vi "Local Tracking.vi"(4 "Offset Home 2 RCM":dbl[](array[numeric])=[0.0, 0.0, 0.0, 0.0], 5 "Trajectory Cluster":T1, 6 "PID Cluster":T4={"L1 to L4 PID Cluster"={"L1 PID Gains"={"Kp"=0.005, "Kd"=0.5, "Ki"=0.0005}, "L2 PID Gains"={"Kp"=0.01, "Kd"=1.0, "Ki"=0.005}, "L3 PID Gains"={"Kp"=0.05, "Kd"=1.0, "Ki"=0.0005}, "L4 PID Gains"={"Kp"=0.1, "Kd"=0.1, "Ki"=0.0005}}, "Stage PID Cluster"={"Stage Z PID"={"Kp"=0.0005, "Kd"=0.001, "Ki"=0.0}, "Stage Y PID"={"Kp"=0.0003, "Kd"=0.01, "Ki"=0.0}, "Stage X PID"={"Kp"=0.0003, "Kd"=0.01, "Ki"=0.0}}, "OCT Z PID Gains"={"Kp"=0.0003, "Kd"=0.0001, "Ki"=0.01}}, 7 "No. Cycles":u8=1, 8 "error in":errorcluster, 10 "Prev Posit Cluster":T3={"Prev L1 to L4 Posit"=[-0.5319, -0.035669172703475985, -2.0566170657346783, 0.9099264705882353], "Prev Stage Posit"=[6.002553885707208, 5.996566124542428, 5.995469940427586], "Prev OCT Z Posit"=-0.0}, 11 "FPGA VI Reference In":refnum<k20>) -> (0 "error out":errorcluster, 2 "Last Posit Cluster":T2={"Last L1 to L4 Posit"=[0.0, 0.0, 0.0, 0.0], "Last Stage Posit"=[6.0, 6.0, 6.0], "Last OCT Z Posit"=0.0}, 3 "FPGA VI Reference Out":refnum<k20>)   [LabVIEW 2016]
uses:
  <vilib>/Platform/TimedLoop/XDataNode/timing_clust.ctl
  <vilib>/Platform/TimedLoop/XDataNode/nitl_modes.ctl
  <vilib>/Platform/TimedLoop/XDataNode/wakeup.ctl
  Global Variables.vi
  <vilib>/platform/TimedLoop/XDataNode/XDataNode.xnode
  <vilib>/Platform/TimedLoop/XDataNode/XDNodeRunTimeDep.lvlib
  Library/KevinLibraryAll/labview/KevLib01.lvlib
panel:
  out "In Servo Loop":bool
  out "Loading Finished":bool
  # "e"
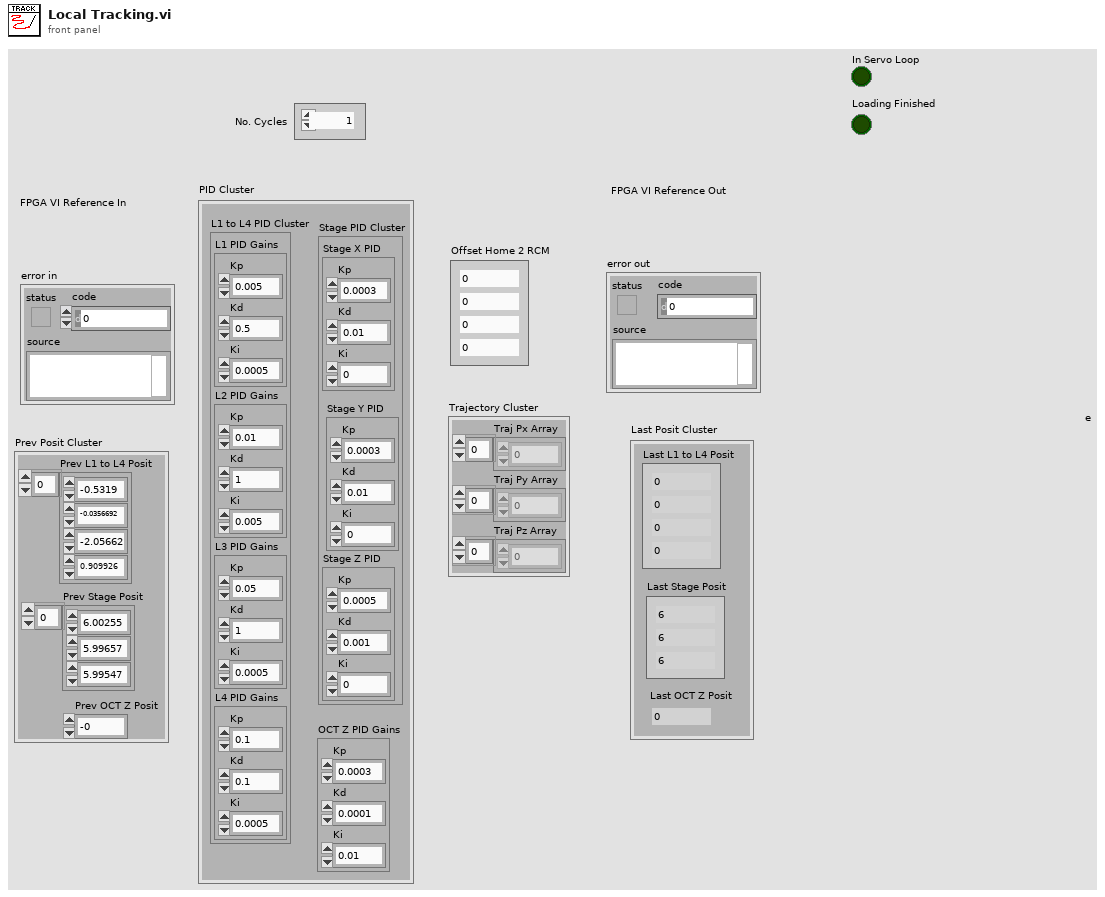
[diagram p1: front panel]
types:
  T1 = cluster{"Traj Px Array":dbl[], "Traj Py Array":dbl[], "Traj Pz Array":dbl[]}
  T2 = cluster{"Last L1 to L4 Posit":dbl[], "Last Stage Posit":dbl[], "Last OCT Z Posit":dbl}
  T3 = cluster{"Prev L1 to L4 Posit":dbl[], "Prev Stage Posit":dbl[], "Prev OCT Z Posit":dbl}
  T4 = cluster{"L1 to L4 PID Cluster":cluster{"L1 PID Gains":cluster{"Kp":dbl, "Kd":dbl, "Ki":dbl}, "L2 PID Gains":cluster{"Kp":dbl, "Kd":dbl, "Ki":dbl}, "L3 PID Gains":cluster{"Kp":dbl, "Kd":dbl, "Ki":dbl}, "L4 PID Gains":cluster{"Kp":dbl, "Kd":dbl, "Ki":dbl}}, "Stage PID Cluster":cluster{"Stage Z PID":cluster{"Kp":dbl, "Kd":dbl, "Ki":dbl}, "Stage Y PID":cluster{"Kp":dbl, "Kd":dbl, "Ki":dbl}, "Stage X PID":cluster{"Kp":dbl, "Kd":dbl, "Ki":dbl}}, "OCT Z PID Gains":cluster{"Kp":dbl, "Kd":dbl, "Ki":dbl}}
  T5 = typedef "XDNodeRunTimeDep.lvlib/timing_clust.ctl" = cluster{"Expected End [f-1]":u64, "Actual End [f-1]":u64, "Finished Late? [f-1]":bool, "Expected End [i-1]":u64, "Actual End [i-1]":u64, "Finished Late? [i-1]":bool, "Expected Start [i]":u64, "Actual Start [i]":u64, "Expected Start [f]":u64, "Actual Start [f]":u64, "Source Name":string, "Structure Name":string, "Period":i64, "Deadline":i64, "Offset":i64, "Start":i64, "Priority":i32, "Timeout":i32, "Mode":T6, "Wakeup Reason":T7, "Error":errorcluster, "Source Type":string, "Secondary Source Type":string, "Global End Time":u64, "Global Start Time":u64, "Frame Duration":u64, "Iteration Duration":u64, "Assigned CPU":i32, "I/O Scan Engine Mode":u32}
  T6 = typedef "XDNodeRunTimeDep.lvlib/nitl_modes.ctl" = enum32{"No Change", "Process missed periods, maintain original phase", "Discard missed periods, maintain original phase", "Process missed periods, ignore original phase", "Discard missed periods, ignore original phase"}
  T7 = typedef "XDNodeRunTimeDep.lvlib/wakeup.ctl" = enum32{"Normal", "Aborted", "Asynchronous wakeup", "Timing source error", "Timed loop error", "Timeout"}
  T8 = cluster{"L1 PID Gains":cluster{"Kp":dbl, "Kd":dbl, "Ki":dbl}, "L2 PID Gains":cluster{"Kp":dbl, "Kd":dbl, "Ki":dbl}, "L3 PID Gains":cluster{"Kp":dbl, "Kd":dbl, "Ki":dbl}, "L4 PID Gains":cluster{"Kp":dbl, "Kd":dbl, "Ki":dbl}}
  T9 = cluster{"Stage Z PID":cluster{"Kp":dbl, "Kd":dbl, "Ki":dbl}, "Stage Y PID":cluster{"Kp":dbl, "Kd":dbl, "Ki":dbl}, "Stage X PID":cluster{"Kp":dbl, "Kd":dbl, "Ki":dbl}}
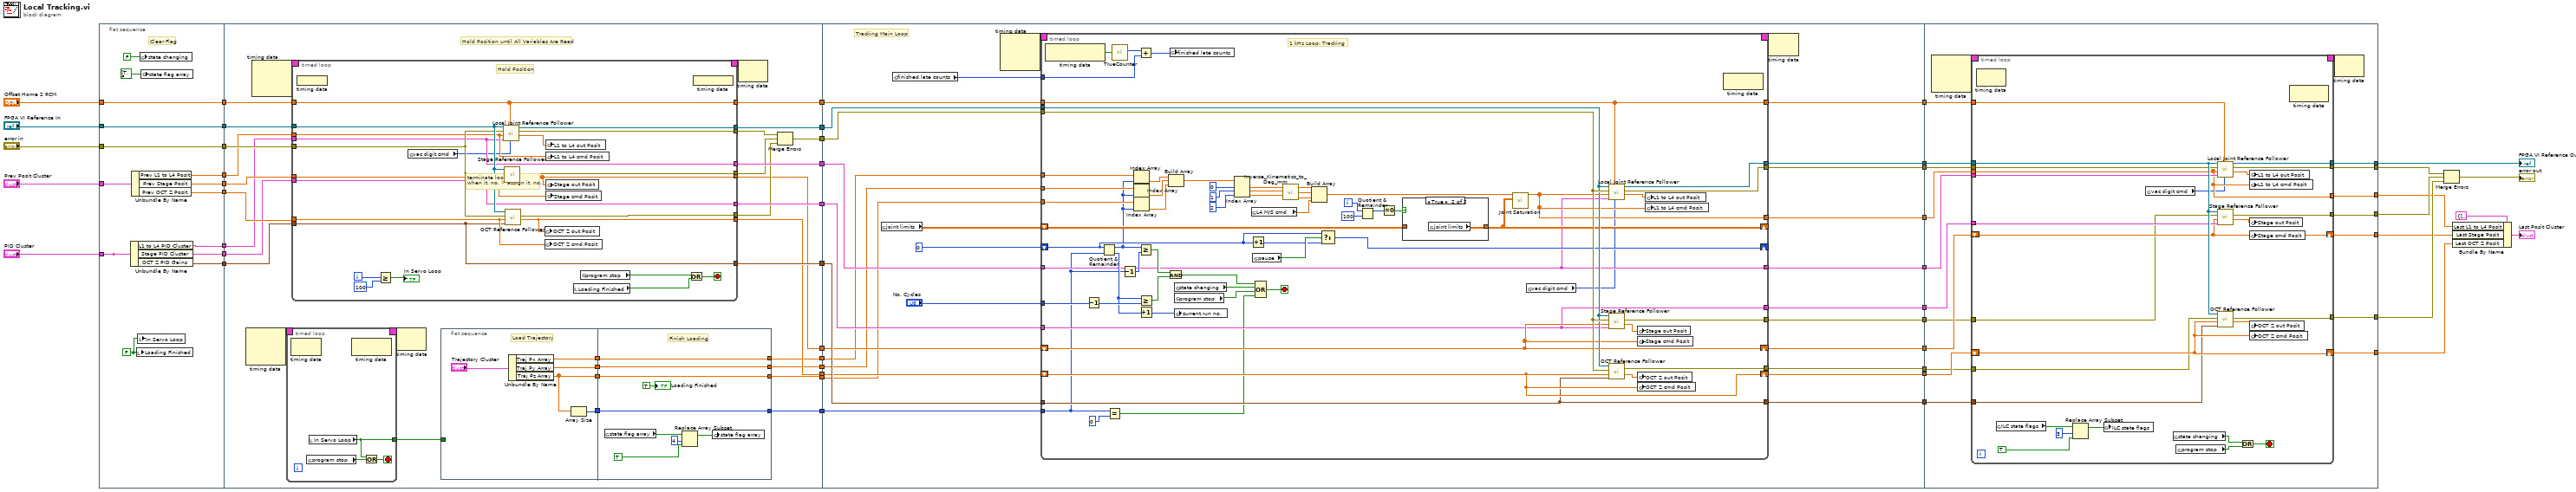
[diagram p0: block diagram]
diagram:
  n1 = flat-sequence {
    tunnel: [w59] -> w47
    tunnel: "FPGA VI Reference In" -> [w59]
    tunnel: "error in" -> [w58]
    tunnel: [w58] -> w44
    tunnel: "Prev Posit Cluster" -> [w57]
    tunnel: [w56] -> _
    tunnel: "PID Cluster" -> [w56]
    tunnel: [w55] -> w41
    tunnel: [w54] -> w40
    tunnel: [w53] -> w39
    tunnel: [w52] -> w38
    tunnel: [w51] -> w37
    tunnel: "Offset Home 2 RCM" -> [w51]
    tunnel: [w50] -> w32
    tunnel: [w48] -> w23
    tunnel: w47 -> [w94]
    tunnel: w44 -> [w93]
    tunnel: w41 -> [w92]
    tunnel: w40 -> [w91]
    tunnel: w39 -> [w90]
    tunnel: w38 -> [w89]
    tunnel: w37 -> [w88]
    tunnel: [w87] -> w35
    tunnel: [w86] -> w34
    tunnel: [w85] -> w33
    tunnel: w32 -> [w84]
    tunnel: [w83] -> w31
    tunnel: [w82] -> w30
    tunnel: [w81] -> w29
    tunnel: w23 -> [w80]
    tunnel: [w74] -> w22
    tunnel: [w73] -> w21
    tunnel: [w66] -> w20
    tunnel: [w65] -> w19
    tunnel: [w64] -> w18
    tunnel: [w62] -> w17
    tunnel: w35 -> [w169]
    tunnel: w34 -> [w154]
    tunnel: w33 -> [w168]
    tunnel: w31 -> [w166]
    tunnel: w30 -> [w165]
    tunnel: w29 -> [w164]
    tunnel: w22 -> [w156]
    tunnel: w21 -> [w155]
    tunnel: w20 -> [w153]
    tunnel: w19 -> [w152]
    tunnel: w18 -> [w151]
    tunnel: w17 -> [w143]
    tunnel: [w163] -> w16
    tunnel: [w162] -> w15
    tunnel: [w161] -> w14
    tunnel: [w160] -> w13
    tunnel: [w159] -> w12
    tunnel: [w158] -> w11
    tunnel: [w157] -> w10
    tunnel: [w147] -> w9
    tunnel: [w146] -> w8
    tunnel: [w145] -> w7
    tunnel: [w144] -> w6
    tunnel: [w252] -> w24
    tunnel: [w258] -> w2
    tunnel: [w253] -> w3
    tunnel: [w245] -> w5
    tunnel: [w246] -> w25
    tunnel: w16 -> [w250]
    tunnel: w15 -> [w249]
    tunnel: w14 -> [w254]
    tunnel: w13 -> [w256]
    tunnel: w12 -> [w259]
    tunnel: w11 -> [w255]
    tunnel: w10 -> [w257]
    tunnel: w9 -> [w260]
    tunnel: w8 -> [w251]
    tunnel: w7 -> [w248]
    tunnel: w6 -> [w247]
    tunnel: [w244] -> w4
    tunnel: [w243] -> w1
    frame #0 {
      w49 = FALSE ("Loading Finished")
      # "Clear Flag"
      n2 = Unbundle By Name(w56) -> ("L1 to L4 PID Cluster"=w52:T8, "Stage PID Cluster"=w50:T9, "OCT Z PID Gains"=w55:cluster{"Kp":dbl, "Kd":dbl, "Ki":dbl})
      n3 = Unbundle By Name(w57) -> ("Prev L1 to L4 Posit"=w48:dbl[], "Prev Stage Posit"=w54:dbl[], "Prev OCT Z Posit"=w53:dbl)
      n4 = local write "Loading Finished"(w49) -> ()
      n5 = local write "In Servo Loop"(w49) -> ()
      n6 = global write "Global Variables.vi" "state changing"(FALSE ("state changing")) -> ()
      n7 = global write "Global Variables.vi" "state flag array"(bool[] [TRUE, FALSE, FALSE, FALSE, FALSE, FALSE, FALSE, FALSE, FALSE] ("state flag array")) -> ()
    }
    frame #1 {
      # "terminate loop\nwhen it. no. > assign it. no."
      # "Hold Position until All Variables Are Read"
      n8 = node-c288() -> (w72:T5)  [unwired: 3 in]
      n9 = node-c288() -> (w79:T5)  [unwired: 3 in]
      n10 = timed-loop {
        timing: w72 -> [_]
        timing-out: [_] -> w71
        tunnel: [w109] -> w70
        stop <- w111 stop-if-true
        n11 = node-c288() -> ()  [unwired: 1 in, 1 out]
        n12 = global read "Global Variables.vi" "program stop"() -> (w110:bool)
        n13 = local read "In Servo Loop"() -> (w109:bool)
        n14 = node-c288() -> ()  [unwired: 1 in, 1 out]
        n15 = Or(x=w109, y=w110) -> (x .or. y?=w111:bool)
      }
      n16 = timed-loop {
        timing: w79 -> [_]
        timing-out: [_] -> w78
        tunnel: [w134] -> w74
        tunnel: [w133] -> w73
        tunnel: [w132] -> w87
        tunnel: [w131] -> w77
        tunnel: [w130] -> w76
        tunnel: [w129] -> w75
        tunnel: w94 -> [w128]
        tunnel: w93 -> [w127]
        tunnel: w92 -> [w122]
        tunnel: w80 -> [w125]
        tunnel: w91 -> [w126]
        tunnel: w90 -> [w124]
        tunnel: w89 -> [w120]
        tunnel: w88 -> [w123]
        tunnel: [w123] -> w86
        tunnel: w84 -> [w121]
        tunnel: [w122] -> w81
        tunnel: [w121] -> w82
        tunnel: [w120] -> w83
        i -> [w119]
        stop <- w138 stop-if-true
        # "Hold Position"
        n17 = node-c288 ("Output Node")() -> ()  [unwired: 1 in]
        n18 = Greater Or Equal?(x=w119, y=100) -> (x >= y?=→"In Servo Loop":bool)
        n19 = global read "Global Variables.vi" "vac digit cmd"() -> (w116:i8)
        n20 = call "Local Joint Reference Follower.vi"("Digital Cmd [0-78]"=w116, "Offset Home2RCM [deg/mm]"=w123, "PID Ctrl Cluster"=w120, "Ref Array [deg/mm]"=w125, "error in"=w127, "FPGA VI Reference In"=w128) -> ("Output Posit Array [deg/mm]"=w135:dbl[], "error out"=w131:errorcluster, "FPGA VI Reference Out"=w132:refnum<k20>)  [unwired: 3 in]
        n21 = call "Stage Reference Follower.vi"("Stage PID Cluster"=w121, "Stage cmd Posit [mm]"=w126, "error in"=w127, "FPGA VI Reference In"=w128) -> ("Stage out Posit [mm]"=w134:dbl[], "error out"=w130:errorcluster)  [unwired: 5 in, 1 out]
        n22 = call "OCT Reference Follower.vi"("OCT Z PID Gains"=w122, "OCT  Z cmd Posit [mm]"=w124, "error in"=w127, "FPGA VI Reference In"=w128) -> ("OCT  Z out Posit [mm]"=w133:dbl, "error out"=w129:errorcluster)  [unwired: 5 in, 1 out]
        n23 = global write "Global Variables.vi" "OCT Z out Posit"(w133) -> ()
        n24 = global write "Global Variables.vi" "OCT Z cmd Posit"(w124) -> ()
        n25 = global write "Global Variables.vi" "L1 to L4 out Posit"(w135) -> ()
        n26 = global write "Global Variables.vi" "L1 to L4 cmd Posit"(w125) -> ()
        n27 = global write "Global Variables.vi" "Stage out Posit"(w134) -> ()
        n28 = global write "Global Variables.vi" "Stage cmd Posit"(w126) -> ()
        n29 = local read "Loading Finished"() -> (w137:bool)
        n30 = global read "Global Variables.vi" "program stop"() -> (w136:bool)
        n31 = Or(x=w136, y=w137) -> (x .or. y?=w138:bool)
        n32 = node-c288() -> ()  [unwired: 1 out]
      }
      n33 = node-c288(w71) -> ()  [unwired: 1 out]
      n34 = flat-sequence {
        tunnel: w70 -> [_]
        tunnel: [w98] -> w69
        tunnel: [w97] -> w68
        tunnel: [w96] -> w67
        tunnel: [w95] -> w63
        tunnel: w69 -> [w105]
        tunnel: w68 -> [w106]
        tunnel: w67 -> [w107]
        tunnel: [w107] -> w66
        tunnel: [w106] -> w65
        tunnel: [w105] -> w64
        tunnel: w63 -> [w104]
        tunnel: [w104] -> w62
        frame #0 {
          # "Load Trajectory"
          n35 = Unbundle By Name("Trajectory Cluster") -> ("Traj Px Array"=w96:dbl[], "Traj Py Array"=w97:dbl[], "Traj Pz Array"=w98:dbl[])
          n36 = Array Size(array=w98) -> (size(s)=w95:i32)
        }
        frame #1 {
          # "Finish Loading"
          n37 = global read "Global Variables.vi" "state flag array"() -> (w101:bool[])
          n38 = Replace Array Subset(array=w101, new element=TRUE ("new element/subarray"), index=4) -> (w100:bool[])
          n39 = global write "Global Variables.vi" "state flag array"(w100) -> ()
          "Loading Finished" <- TRUE ("Loading Finished")
        }
      }
      n40 = node-c288(w78) -> ()  [unwired: 1 out]
      n41 = Merge Errors(w77, w76, w75) -> (w85:errorcluster)
    }
    frame #2 {
      # "Tracking Main Loop"
      n42 = global read "Global Variables.vi" "joint limits"() -> (w148:dbl[][])
      n43 = global read "Global Variables.vi" "finished late counts"() -> (w167:u16)
      n44 = node-c288() -> (w171:T5)  [unwired: 3 in]
      n45 = timed-loop {
        timing: w171 -> [_]
        timing-out: [_] -> w170
        tunnel: w153 -> [w235]
        tunnel: w152 -> [w234]
        tunnel: w151 -> [w218]
        tunnel: w169 -> [w230]
        tunnel: w154 -> [w183]
        tunnel: w168 -> [w231]
        tunnel: [w232] -> w163
        tunnel: w166 -> [w180]
        tunnel: w167 -> [w226]
        tunnel: w165 -> [w182]
        tunnel: w164 -> [w181]
        shift-right: [w185] -> w158
        shift-left: w156 -> [w185]
        shift-right: [w184] -> w157
        shift-left: w155 -> [w184]
        tunnel: [w223] -> w161
        tunnel: [w222] -> w160
        tunnel: [w221] -> w162
        tunnel: [w175] -> w159
        tunnel: "No. Cycles" -> [w194]
        shift-right: [w192] -> _
        shift-left: 0 ("No. Cycles") -> [w179]
        tunnel: w143 -> [w178]
        shift-right: [w187] -> _
        shift-left: w148 -> [w186]
        tunnel: [w183] -> w147
        tunnel: [w182] -> w144
        tunnel: [w181] -> w146
        tunnel: [w180] -> w145
        i -> [w191]
        stop <- w199 stop-if-true
        # "Hold Position if not Engaged"
        # "1 kHz Loop: Tracking"
        n46 = node-c288() -> (w229:bool)  [unwired: 1 in]
        n47 = Decrement(x=w194) -> (x-1=w205:u8)
        n48 = Quotient & Remainder(x=w179, y=w178) -> (x-y*floor(x/y)=w173:i32, floor(x/y)=w193:i32)
        n49 = Equal?(x=w178, y=0) -> (x = y?=w176:bool)
        n50 = call "TrueCounter.vi"("True?"=w229) -> ("True Count"=w227:u16)  [unwired: 10 in]
        n51 = Decrement(x=w178) -> (x-1=w206:i32)
        n52 = Index Array(array=w235, index=w173) -> (element=w210:dbl)
        n53 = Index Array(array=w234, index=w173) -> (element=w209:dbl)
        n54 = Index Array(array=w218, index=w173) -> (element=w208:dbl)
        n55 = Add(x=w227, y=w226) -> (x+y=w228:u16)
        n56 = Greater Or Equal?(x=w173, y=w206) -> (x >= y?=w204:bool)
        n57 = Greater Or Equal?(x=w193, y=w205) -> (x >= y?=w203:bool)
        n58 = Increment(x=w193) -> (x+1=w195:i32)
        n59 = And(x=w204, y=w203) -> (x .and. y?=w202:bool)
        n60 = Build Array(w210, w209, w208) -> (w207:dbl[])
        n61 = global write "Global Variables.vi" "finished late counts"(w228) -> ()
        n62 = global read "Global Variables.vi" "state changing"() -> (w201:bool)
        n63 = global read "Global Variables.vi" "program stop"() -> (w200:bool)
        n64 = global write "Global Variables.vi" "current run no."(w195) -> ()
        n65 = Index Array(array=w207, index #1=0 ("index"), index #2=1 ("index"), index #3=2 ("index")) -> (element #1=w213:dbl, element #2=w212:dbl, element #3=w211:dbl)
        n66 = Increment(x=w179) -> (x+1=w196:i32)
        n67 = global read "Global Variables.vi" "L4 M/S cmd"() -> (w198:dbl)
        n68 = global read "Global Variables.vi" "pause"() -> (w197:bool)
        n69 = Compound Arithmetic op=OR(w202, w201, w200, w176) -> (w199:bool)
        n70 = call "Inverse_Kinematics_to_Deg_mm.vi"("pz"=w211, "py"=w212, "px"=w213) -> ("L3 [mm]"=w219:dbl, "L2 [deg]"=w220:dbl, "L1 [deg]"=w233:dbl)
        n71 = Build Array(w233, w220, w219, w198) -> (w217:dbl[])
        n72 = Select(t=w179, s=w197, f=w196) -> (s? t:f=w192:i32)
        n73 = Quotient & Remainder(x=w191, y=100) -> (x-y*floor(x/y)=w189:i32)  [unwired: 1 out]
        n74 = Equal To 0?(x=w189) -> (x = 0?=w188:bool)
        n75 = case shown="True" w188 {
          tunnel: [w236 w237] -> w187
          tunnel: w186 -> [w236 _]
          frame False {
          }
          frame True {
            n76 = global read "Global Variables.vi" "joint limits"() -> (w237:dbl[][])
          }
        }
        n77 = call "Joint Saturation.vi"("Joint Bounds [Deg/mm]"=w187, "Ref Array [Deg/mm]"=w217) -> ("Sat Ref Array [Deg/mm]"=w175:dbl[])  [unwired: 9 in]
        n78 = global read "Global Variables.vi" "vac digit cmd"() -> (w172:i8)
        n79 = call "Local Joint Reference Follower.vi"("Digital Cmd [0-78]"=w172, "Offset Home2RCM [deg/mm]"=w183, "PID Ctrl Cluster"=w180, "Ref Array [deg/mm]"=w175, "error in"=w231, "FPGA VI Reference In"=w230) -> ("Output Posit Array [deg/mm]"=w174:dbl[], "error out"=w221:errorcluster, "FPGA VI Reference Out"=w232:refnum<k20>)  [unwired: 3 in]
        n80 = call "Stage Reference Follower.vi"("Stage PID Cluster"=w182, "Stage cmd Posit [mm]"=w185, "error in"=w231, "FPGA VI Reference In"=w230) -> ("Stage out Posit [mm]"=w225:dbl[], "error out"=w223:errorcluster)  [unwired: 5 in, 1 out]
        n81 = call "OCT Reference Follower.vi"("OCT Z PID Gains"=w181, "OCT  Z cmd Posit [mm]"=w184, "error in"=w231, "FPGA VI Reference In"=w230) -> ("OCT  Z out Posit [mm]"=w224:dbl, "error out"=w222:errorcluster)  [unwired: 5 in, 1 out]
        n82 = global write "Global Variables.vi" "Stage out Posit"(w225) -> ()
        n83 = global write "Global Variables.vi" "Stage cmd Posit"(w185) -> ()
        n84 = global write "Global Variables.vi" "OCT Z out Posit"(w224) -> ()
        n85 = global write "Global Variables.vi" "OCT Z cmd Posit"(w184) -> ()
        n86 = global write "Global Variables.vi" "L1 to L4 out Posit"(w174) -> ()
        n87 = global write "Global Variables.vi" "L1 to L4 cmd Posit"(w175) -> ()
        n88 = node-c288() -> ()  [unwired: 1 in, 1 out]
      }
      n89 = node-c288(w170) -> ()  [unwired: 1 out]
    }
    frame #3 {
      n90 = node-c288() -> (w262:T5)  [unwired: 3 in]
      n91 = timed-loop {
        timing: w262 -> [_]
        timing-out: [_] -> w261
        tunnel: w250 -> [w285]
        tunnel: w248 -> [w284]
        tunnel: w247 -> [w283]
        tunnel: w256 -> [w270]
        tunnel: w259 -> [w274]
        tunnel: w260 -> [w282]
        tunnel: [w281] -> w246
        tunnel: [w280] -> w245
        tunnel: [w274] -> w258
        tunnel: [w276] -> w244
        tunnel: [w275] -> w253
        shift-right: [w273] -> w243
        shift-left: w255 -> [w273]
        shift-right: [w272] -> w252
        shift-left: w257 -> [w272]
        tunnel: w254 -> [w271]
        tunnel: w251 -> [w269]
        tunnel: w249 -> [w268]
        stop <- w288 stop-if-true
        n92 = node-c288() -> ()  [unwired: 1 in, 1 out]
        n93 = global read "Global Variables.vi" "ILC state flags"() -> (w266:bool[])
        n94 = Replace Array Subset(array=w266, new element=TRUE ("new element/subarray"), index=3) -> (w265:bool[])
        n95 = global write "Global Variables.vi" "ILC state flags"(w265) -> ()
        n96 = global read "Global Variables.vi" "vac digit cmd"() -> (w263:i8)
        n97 = global read "Global Variables.vi" "state changing"() -> (w287:bool)
        n98 = global read "Global Variables.vi" "program stop"() -> (w286:bool)
        n99 = call "Local Joint Reference Follower.vi"("Digital Cmd [0-78]"=w263, "Offset Home2RCM [deg/mm]"=w282, "PID Ctrl Cluster"=w284, "Ref Array [deg/mm]"=w274, "error in"=w268, "FPGA VI Reference In"=w285) -> ("Output Posit Array [deg/mm]"=w279:dbl[], "error out"=w280:errorcluster, "FPGA VI Reference Out"=w281:refnum<k20>)  [unwired: 3 in]
        n100 = call "Stage Reference Follower.vi"("Stage PID Cluster"=w283, "Stage cmd Posit [mm]"=w273, "error in"=w271, "FPGA VI Reference In"=w285) -> ("Stage out Posit [mm]"=w278:dbl[], "error out"=w276:errorcluster)  [unwired: 5 in, 1 out]
        n101 = call "OCT Reference Follower.vi"("OCT Z PID Gains"=w269, "OCT  Z cmd Posit [mm]"=w272, "error in"=w270, "FPGA VI Reference In"=w285) -> ("OCT  Z out Posit [mm]"=w277:dbl, "error out"=w275:errorcluster)  [unwired: 5 in, 1 out]
        n102 = Or(x=w287, y=w286) -> (x .or. y?=w288:bool)
        n103 = global write "Global Variables.vi" "L1 to L4 out Posit"(w279) -> ()
        n104 = global write "Global Variables.vi" "L1 to L4 cmd Posit"(w274) -> ()
        n105 = global write "Global Variables.vi" "Stage out Posit"(w278) -> ()
        n106 = global write "Global Variables.vi" "Stage cmd Posit"(w273) -> ()
        n107 = global write "Global Variables.vi" "OCT Z out Posit"(w277) -> ()
        n108 = global write "Global Variables.vi" "OCT Z cmd Posit"(w272) -> ()
        n109 = node-c288() -> ()  [unwired: 1 in, 1 out]
      }
      n110 = node-c288(w261) -> ()  [unwired: 1 out]
    }
  }
  n111 = Merge Errors(w5, w4, w3) -> (→"error out":errorcluster)
  n112 = Bundle By Name(cluster=T2 {"Last L1 to L4 Posit"=[0.0, 0.0, 0.0, 0.0], "Last Stage Posit"=[6.0, 6.0, 6.0], "Last OCT Z Posit"=0.0} ("Last Posit Cluster 2"), "Last L1 to L4 Posit"=w2, "Last Stage Posit"=w1, "Last OCT Z Posit"=w24) -> (→"Last Posit Cluster":T2)
  "FPGA VI Reference Out" <- w25
